vi "analyse.vi"(8 "error in (no error)":errorcluster, 11 "DL090623TwoDAnalyser in":refnum<class "AnalyserDL090623TwoD.lvclass">) -> (0 "error out":errorcluster, 3 "DL090623TwoDAnalyser out":refnum<class "AnalyserDL090623TwoD.lvclass">)   [LabVIEW 2010, in "AnalyserDL090623TwoD.lvclass"]
uses:
  AnalyserDL090623TwoD.lvclass
  common/classes/Image/Image/Image.lvclass
  AnalyserDL090623TwoD.lvclass/AnalyserDL090623TwoD.ctl
  TraceProcessor/GenericTraceProcessor/GenericTraceProcessor/GenericTraceProcessor.lvclass
  common/classes/ErrorController/ErrorController/class_data.vi
  <vilib>/vision/NI_Vision_Development_Module.lvlib
  common/classes/ErrorController/ErrorController/ErrorController.lvclass
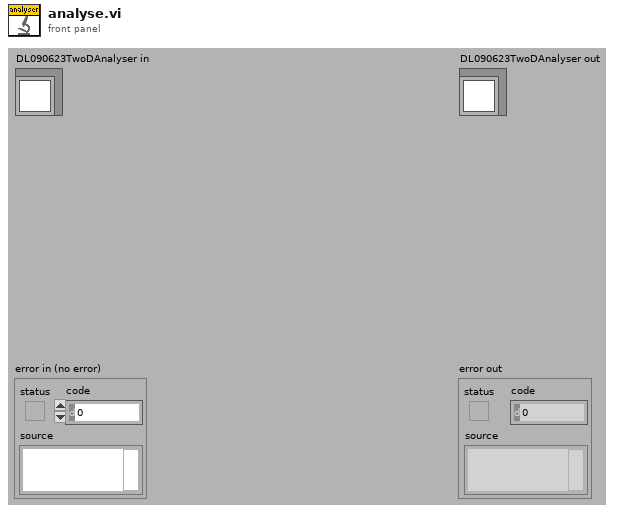
[diagram p1: front panel]
types:
  T1 = typedef "ROI Descriptor" = cluster{"Global Rectangle":i32[], "Contours":cluster{"ID":enum32{"External", "Internal"}, "Type":u32, "Coordinates":i32[]}[]}
  T2 = typedef "IMAQ Image.ctl" = refnum<image>
  T3 = cluster{"Min":sgl, "Max":sgl, "Mean":sgl, "Std Dev":sgl, "Count":i32}
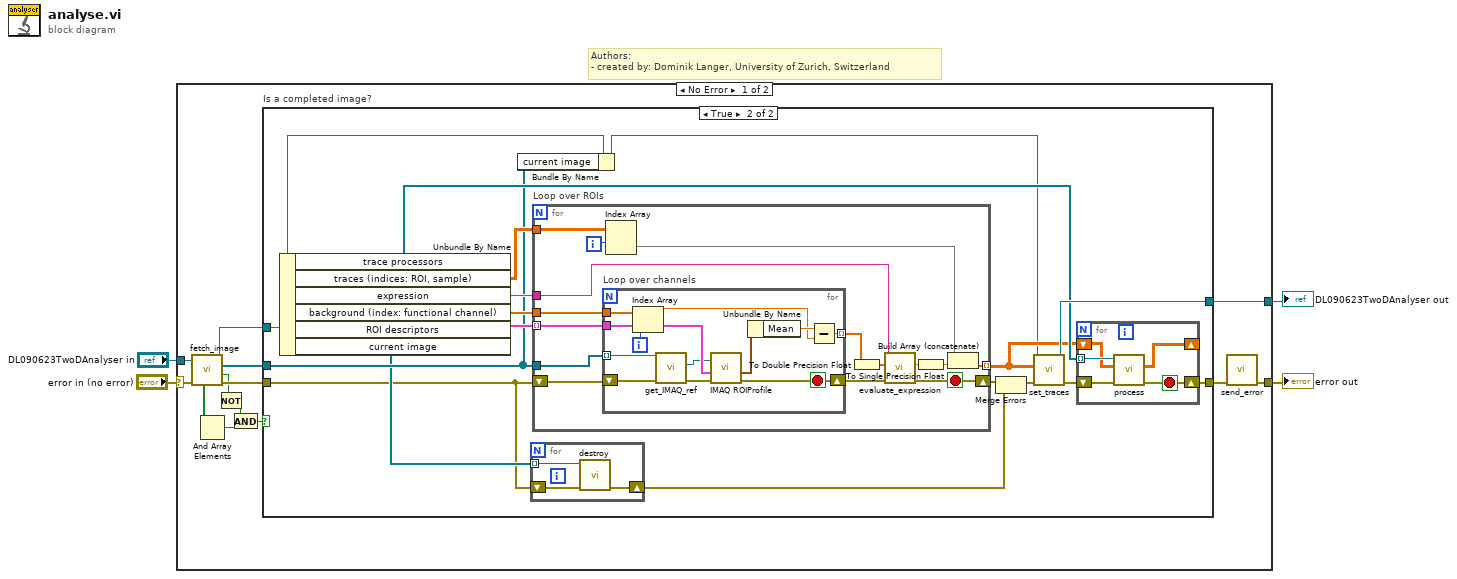
[diagram p0: block diagram]
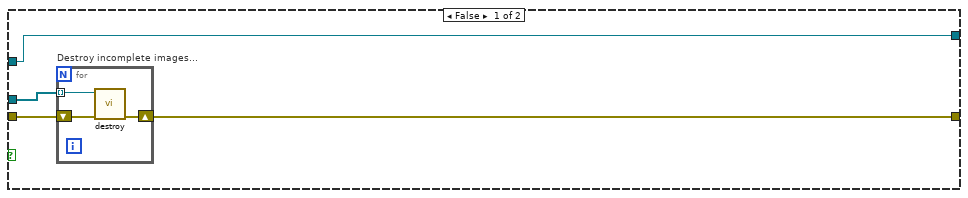
[diagram p2: hidden frame]
diagram:
  # "Authors: \n- created by: Dominik Langer, University of Zurich, Switzerland"
  n1 = case shown="No Error" "error in (no error)" {
    selector: "error in (no error)" -> [w16 w78]
    tunnel: [w13 w78] -> w3
    tunnel: [w17 w77] -> w1
    tunnel: "DL090623TwoDAnalyser in" -> [w15 w77]
    frame No Error {
      n2 = call-dynamic "fetch_image.vi"("error in (no error)"=w16, "GenericToplevelComponent in"=w15) -> ("error out"=w12:errorcluster, "channels array empty?"=w5:bool, "image (channels)"=w10:refnum<class "Image.lvclass">[], "GenericToplevelComponent out"=w11:refnum<class "AnalyserDL090623TwoD.lvclass">, "finished?"=w9:bool[])  [unwired: 4 in, 1 out]
      n3 = And Array Elements(Boolean array=w9) -> (logical AND=w8:bool)
      n4 = Not(x=w5) -> (.not. x?=w7:bool)
      n5 = And(x=w7, y=w8) -> (x .and. y?=w6:bool)
      n6 = case "Is a completed image?" shown="True" w6 {
        tunnel: [w21 w38] -> w17
        tunnel: [w19 w33] -> w14
        tunnel: w12 -> [w20 w28]
        tunnel: w11 -> [w21 w32]
        tunnel: w10 -> [w18 w30]
        frame False {
          n7 = for "Destroy incomplete images..." {
            shift-right: [w23] -> w19
            shift-left: w20 -> [w24]
            tunnel: w18 -> [w22] mode=indexing
            n8 = call-dynamic "destroy.vi"("error in (no error)"=w24, "Image in"=w22) -> ("error out"=w23:errorcluster)  [unwired: 8 in, 1 out]
          }
        }
        frame True {
          n9 = Unbundle By Name(w32) -> ("trace processors"=w35:refnum<class "GenericTraceProcessor.lvclass">[], "traces (indices: ROI, sample)"=w37:sgl[][], "expression"=w39:string, "background (index: functional channel)"=w40:sgl[], "ROI descriptors"=w41:T1[], "current image"=w29:refnum<class "Image.lvclass">[])
          n10 = Bundle By Name(cluster=w32, "current image"=w30) -> (w31:refnum<class "AnalyserDL090623TwoD.lvclass">)
          n11 = for {
            shift-right: [w43] -> w27
            shift-left: w28 -> [w44]
            tunnel: w29 -> [w42] mode=indexing
            n12 = call-dynamic "destroy.vi"("error in (no error)"=w44, "Image in"=w42) -> ("error out"=w43:errorcluster)  [unwired: 8 in, 1 out]
          }
          n13 = for "Loop over ROIs" {
            tunnel: w30 -> [w62]
            tunnel: w41 -> [w64] mode=indexing
            tunnel: w40 -> [w61]
            tunnel: w37 -> [w54]
            tunnel: [w58] -> w34 mode=indexing
            tunnel: w39 -> [w55]
            shift-right: [w50] -> w26
            shift-left: w28 -> [w63]
            i -> [w53]
            stop <- w50 stop-if-true
            n14 = for "Loop over channels" {
              tunnel: w64 -> [w75]
              tunnel: w62 -> [w69] mode=indexing
              tunnel: w61 -> [w68]
              tunnel: [w70] -> w51 mode=indexing
              shift-right: [w65] -> w60
              shift-left: w63 -> [w74]
              i -> [w67]
              stop <- w65 stop-if-true
              n15 = Index Array(array=w68, index=w67) -> (element=w66:sgl)
              n16 = call-dynamic "get_IMAQ_ref.vi"("error in (no error)"=w74, "Image.lvclass in"=w69) -> ("error out"=w73:errorcluster, "Image"=w72:T2)  [unwired: 8 out]
              n17 = call "IMAQ ROIProfile"("error in (no error)"=w73, "ROI Descriptor"=w75, "Image"=w72) -> ("ROI Pixel Statistics"=w76:T3, "error out"=w65:errorcluster)  [unwired: 4 out]
              n18 = Unbundle By Name(w76) -> ("Mean"=w71:sgl)
              n19 = Subtract(x=w71, y=w66) -> (x-y=w70:sgl)
            }
            n20 = Index Array(array=w54, index (row)=w53) -> (element=w52:sgl[])  [unwired: 1 in]
            n21 = To Double Precision Float(number=w51) -> (double precision float=w59:dbl[])
            n22 = call "evaluate_expression.vi"("error in (no error)"=w60, "values"=w59, "expression"=w55) -> ("error out"=w50:errorcluster, "result"=w57:dbl)  [unwired: 7 out]
            n23 = To Single Precision Float(number=w57) -> (single precision float=w56:sgl)
            n24 = Build Array (concatenate)(w52, w56) -> (w58:sgl[])
          }
          n25 = Merge Errors(w26, w27) -> (w25:errorcluster)
          n26 = call-dynamic "set_traces.vi"("error in (no error)"=w25, "traces (indices: ROI, sample)"=w34, "DL090623TwoDAnalyser.lvclass in"=w31) -> ("error out"=w36:errorcluster, "DL090623TwoDAnalyser.lvclass out"=w38:refnum<class "AnalyserDL090623TwoD.lvclass">)  [unwired: 7 out]
          n27 = for {
            tunnel: w35 -> [w48] mode=indexing
            shift-right: [w46] -> _
            shift-left: w34 -> [w47]
            shift-right: [w45] -> w33
            shift-left: w36 -> [w49]
            stop <- w45 stop-if-true
            n28 = call-dynamic "process.vi"("error in (no error)"=w49, "input"=w47, "GenericTraceProcessor in"=w48) -> ("error out"=w45:errorcluster, "output"=w46:sgl[][])  [unwired: 7 out]
          }
        }
      }
      n29 = call "send_error.vi"("error in (no error)"=w14) -> ("error out"=w13:errorcluster)  [unwired: 10 in]
    }
    frame Error {
    }
  }
  "error out" <- w3
  "DL090623TwoDAnalyser out" <- w1
